vi "WFM MNGR Add ET Waveform to Database.vi"(8 "error in (no error)":errorcluster, 10 "ET Waveform":T1, 11 "WFM MNGR in":refnum<class "QPA MSMT Waveform Manager.lvclass">) -> (0 "error out":errorcluster, 2 "ET Waveform":T1, 3 "WFM MNGR out":refnum<class "QPA MSMT Waveform Manager.lvclass">)   [LabVIEW 2016, in "QPA MSMT Waveform Manager.lvclass"]
uses:
  QPA MSMT Waveform Manager.lvclass
  Controls/ET Waveform.ctl
  QPA MSMT Waveform Manager.lvclass/QPA MSMT Waveform Manager.ctl
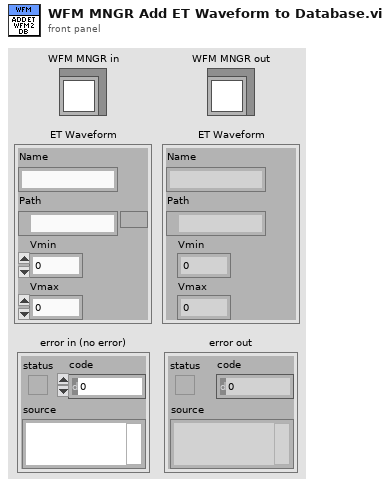
[diagram p1: front panel]
types:
  T1 = typedef "QPA MSMT Waveform Manager.lvclass/ET Waveform.ctl" = cluster{"Name":string, "Path":path, "Vmin":dbl, "Vmax":dbl}
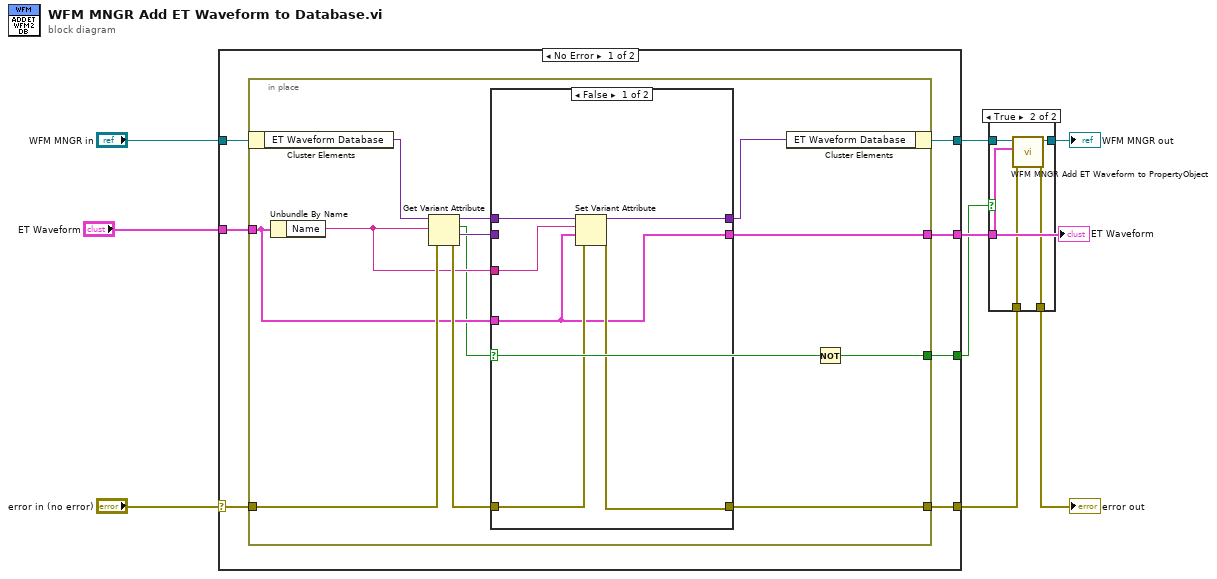
[diagram p0: block diagram]
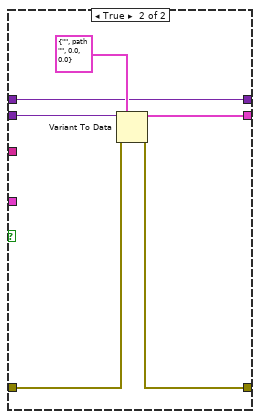
[diagram p3: hidden frame]
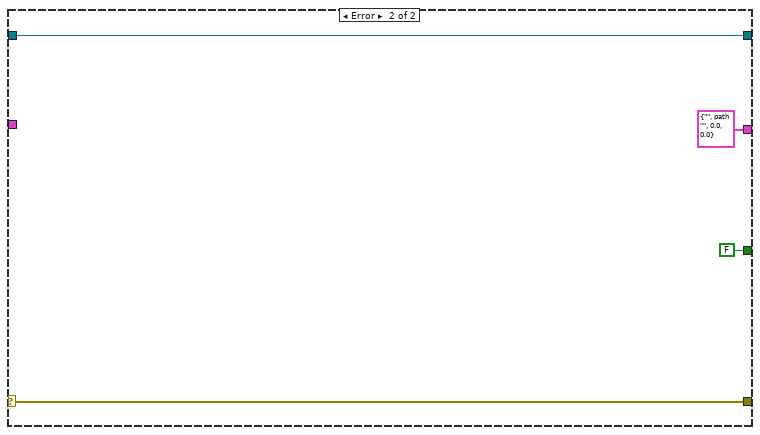
[diagram p4: hidden frame]
diagram:
  n1 = case shown="No Error" "error in (no error)" {
    selector: "error in (no error)" -> [w14 w44]
    tunnel: [w12 w44] -> w3
    tunnel: [w15 w43] -> w7
    tunnel: "WFM MNGR in" -> [w16 w43]
    tunnel: "ET Waveform" -> [w13 _]
    tunnel: [w11 T1 {"Name"="", "Path"=path "", "Vmin"=0.0, "Vmax"=0.0} ("ET Waveform")] -> w2
    tunnel: [w10 FALSE] -> w1
    frame No Error {
      n2 = in-place {
        in-place-border: w14 -> [w27]
        in-place-border: w13 -> [w20]
        in-place-border: [w24] -> w12
        in-place-border: [w23] -> w11
        in-place-border: [w17] -> w10
        n3 = in-place-cluster #1(w16) -> ("ET Waveform Database"=w28:variant)
        n4 = Unbundle By Name(w20) -> ("Name"=w19:string)
        n5 = Get Variant Attribute(Variant=w28, name=w19, error in=w27) -> (duplicate Variant=w22:variant, found=w18:bool, value=w26:variant, error out=w25:errorcluster)  [unwired: 1 in]
        n6 = case shown="False" w18 {
          tunnel: w26 -> [_ w39]
          tunnel: w25 -> [w33 w38]
          tunnel: [w32 w37] -> w24
          tunnel: [w30 w36] -> w23
          tunnel: w22 -> [w34 w35]
          tunnel: [w31 w35] -> w21
          tunnel: w20 -> [w30 _]
          tunnel: w19 -> [w29 _]
          frame False {
            n7 = Set Variant Attribute(Variant=w34, name=w29, value=w30, error in=w33) -> (Variant out=w31:variant, error out=w32:errorcluster)  [unwired: 1 out]
          }
          frame True {
            n8 = Variant To Data(error in=w38, type=T1 {"Name"="", "Path"=path "", "Vmin"=0.0, "Vmax"=0.0} ("ET Waveform"), Variant=w39) -> (data=w36:T1, error out=w37:errorcluster)
          }
        }
        n9 = in-place-cluster #1("ET Waveform Database"=w21) -> (w15:refnum<class "QPA MSMT Waveform Manager.lvclass">)
        n10 = Not(x=w18) -> (.not. x?=w17:bool)
      }
    }
    frame Error {
    }
  }
  "ET Waveform" <- w2
  n11 = case shown="True" w1 {
    tunnel: w7 -> [w46 w51]
    tunnel: [w46 w50] -> w5
    tunnel: [w45 w49] -> w4
    tunnel: w3 -> [w45 w48]
    tunnel: w2 -> [_ w47]
    frame False {
    }
    frame True {
      n12 = call "WFM MNGR Add ET Waveform to PropertyObject.vi"("error in (no error)"=w48, "ET Waveform"=w47, "WFM MNGR in"=w51) -> ("error out"=w49:errorcluster, "WFM MNGR out"=w50:refnum<class "QPA MSMT Waveform Manager.lvclass">)  [unwired: 7 in]
    }
  }
  "error out" <- w4
  "WFM MNGR out" <- w5
